vi "ElevatorSystemV2SetState.vi"(1 "Intake Status":T1, 2 "Scoring Deploy Status":cluster{"State":enum16{"Idle", "Deploy"}}, 3 "Elevator Inputs":T2) -> (0 "Elevator Status":T3)   [LabVIEW 2014]
panel:
  in  "Ready to Index?":bool
  # "Low Height"
  # "High Height"
  # "Elevator Motor"
  # "Elevator Encoder"
  # "Proximity Sensor"
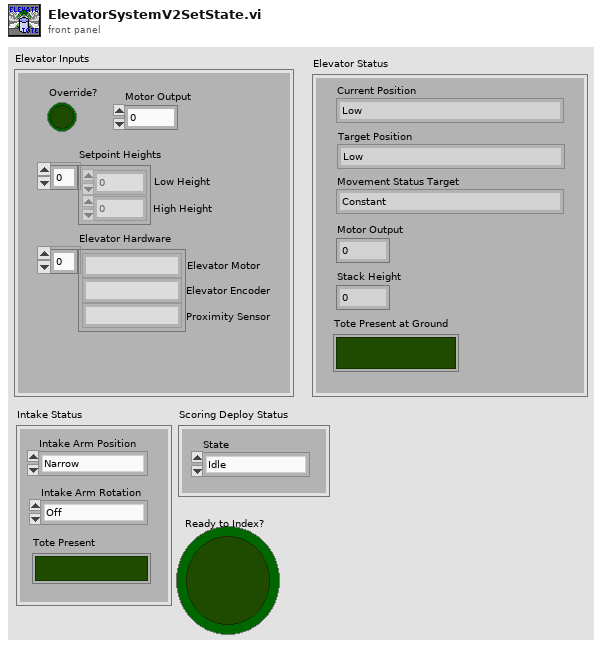
[diagram p1: front panel]
types:
  T1 = cluster{"Intake Arm Position":enum16{"Narrow", "Wide"}, "Intake Arm Rotation":enum16{"Off", "In", "Out", "Rotate Tote"}, "Tote Present":bool}
  T2 = cluster{"Motor Output":dbl, "Override?":bool, "Setpoint Heights":dbl[], "Elevator Hardware":string[]}
  T3 = cluster{"Current Position":enum16{"Low", "High", "Intermediary (Between positions)"}, "Movement Status Target":enum16{"Constant", "Lifting", "Lowering"}, "Stack Height":i32, "Tote Present at Ground":bool, "Target Position":enum16{"Low", "High"}, "Motor Output":dbl}
  T4 = enum16{"Low", "High", "Intermediary (Between positions)"}
  T5 = typedef "WPI_EncoderDevRef.ctl" = cluster{"DevStatus":errorcluster, "EncoderIndex":T6, "CounterIndex":T7, "DistancePerCount":dbl, "Decoding Type":T8}
  T6 = typedef "FPGA_EncoderIdx.ctl" = enum8{"Enc 0", "Enc 1", "Enc 2", "Enc 3", "Enc 4", "Enc 5", "Enc 6", "Enc 7", "Invalid"}
  T7 = typedef "FPGA_CounterCtrSystemIndex.ctl" = enum8{"Ctr 0", "Ctr 1", "Ctr 2", "Ctr 3", "Ctr 4", "Ctr 5", "Ctr 6", "Ctr 7", "Invalid"}
  T8 = typedef "WPI_EncoderType.ctl" = enum16{"1x", "2x", "4x"}
  T9 = typedef "WPI_DigitalInputDevRef.ctl" = cluster{"DevStatus":errorcluster, "DIO Channel":T10, "Controller":T11}
  T10 = typedef "FPGA_DIOChannel.ctl" = enum8{"DIO 0", "DIO 1", "DIO 2", "DIO 3", "DIO 4", "DIO 5", "DIO 6", "DIO 7", "DIO 8", "DIO 9", "DIO MXP 0", "DIO MXP 1", "DIO MXP 2", "DIO MXP 3", "DIO MXP 4", "DIO MXP 5", "DIO MXP 6", "DIO MXP 7", "DIO MXP 8", "DIO MXP 9", "DIO MXP 10", "DIO MXP 11", "DIO MXP 12", "DIO MXP 13", "DIO MXP 14", "DIO MXP 15", "Invalid"}
  T11 = typedef "FPGA_TypedefDigitalModule.ctl" = enum16{"Controller 1"}
  T12 = typedef "WPI_MotorControlDeviceRef.ctl" = cluster{"DeviceStatus":errorcluster, "Type":T13, "PWM":cluster{"Controller":T11, "PWM Channel":T14, "DeadBand":T15}, "CAN":cluster{"Device Number":u8, "Control Mode":T16, "Semaphore":T17, "Max Vout":dbl, "TalonSRX Control Mode":T18}, "Invert":bool, "TransformRef":T19, "InvTransformRef":T19}
  T13 = typedef "WPI_MotorControlType.ctl" = enum16{"PWM", "CAN", "CANTalonSRX"}
  T14 = typedef "FPGA_DIOPWMChannel.ctl" = enum8{"PWM 0", "PWM 1", "PWM 2", "PWM 3", "PWM 4", "PWM 5", "PWM 6", "PWM 7", "PWM 8", "PWM 9", "PWM MXP 0", "PWM MXP 1", "PWM MXP 2", "PWM MXP 3", "PWM MXP 4", "PWM MXP 5", "PWM MXP 6", "PWM MXP 7", "PWM MXP 8", "PWM MXP 9", "Invalid"}
  T15 = typedef "WPI_PWMDeadband.ctl" = cluster{"Name":string, "maxPositivePwm":i32, "minPositivePwm":i32, "centerPwm":i32, "maxNegativePwm":i32, "minNegativePwm":i32, "angularRange":u16}
  T16 = typedef "WPI_CANJaguar_ControlMode.ctl" = enum8{"Percent VBus", "Current", "Speed", "Position", "Voltage"}
  T17 = typedef "Semaphore RefNum" = refnum<k1>
  T18 = typedef "WPI_CANTalonSRX_APIControlMode.ctl" = enum8{"Percent VBus", "Speed", "Position", "Slave", "Unchanged / Invalid"}
  T19 = typedef "WPI_PWMTransform_ConPane.ctl" = refnum<vi>
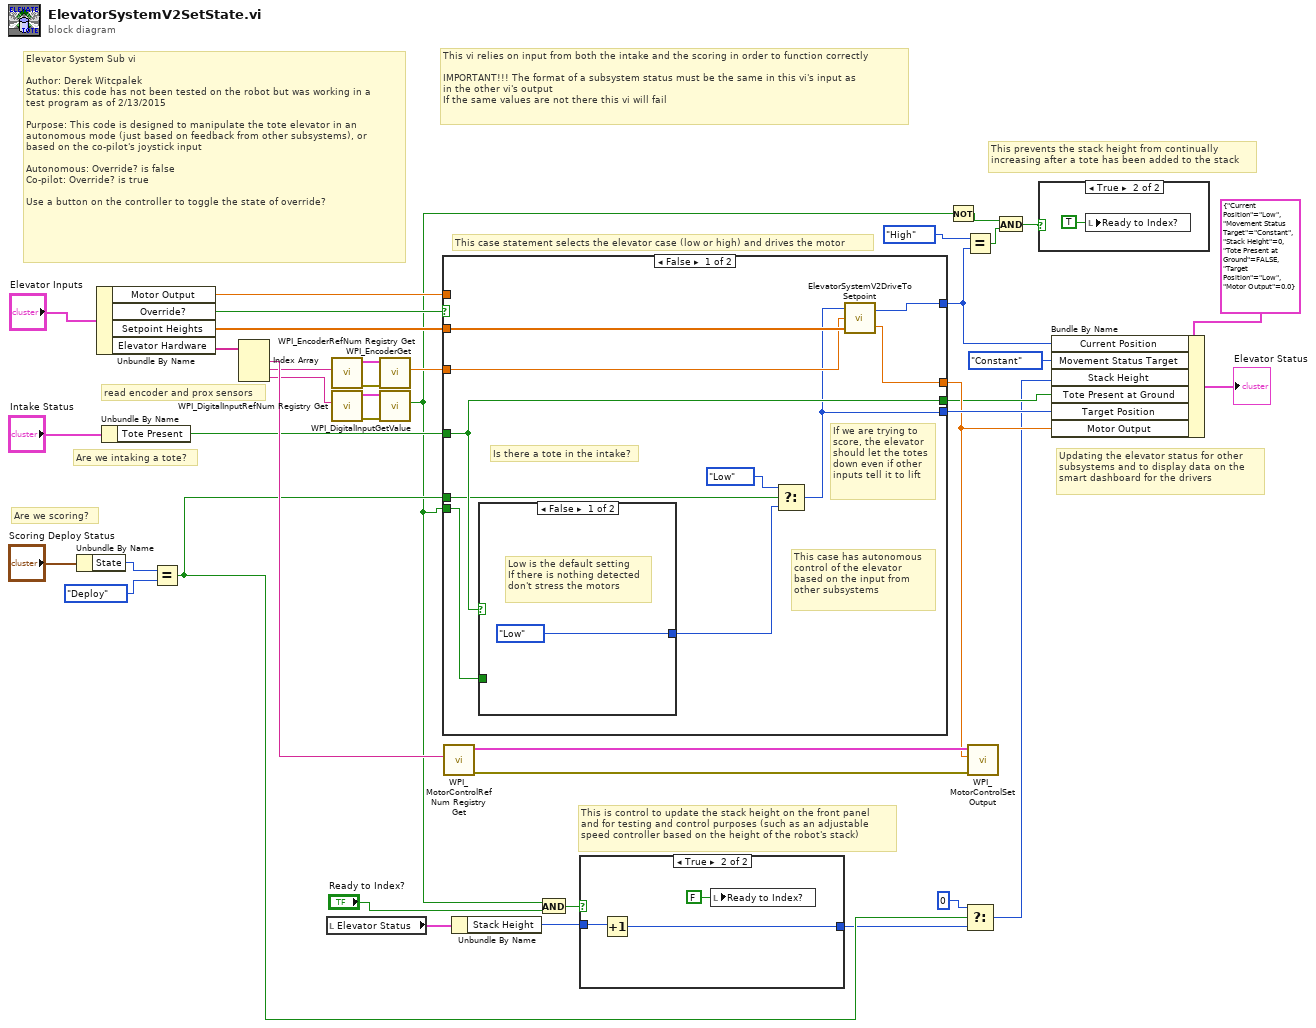
[diagram p0: block diagram]
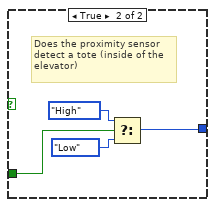
[diagram p4: hidden frame]
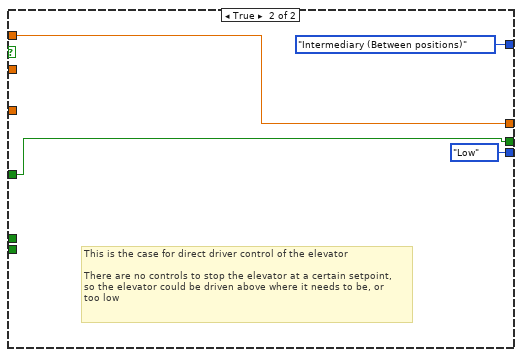
[diagram p5: hidden frame]
diagram:
  # "This vi relies on input from both the intake and the scoring in order to function correctly\n\nIMPORTANT!!! The format of a subsystem status must be the same in this vi's input as\nin the other vi's output\nIf the same values are not there this vi will fail"
  # "Are we intaking a tote?"
  # "Are we scoring?"
  # "read encoder and prox sensors"
  # "Updating the elevator status for other\nsubsystems and to display data on the \nsmart dashboard for the drivers"
  # "This prevents the stack height from continually\nincreasing after a tote has been added to the stack"
  # "This is control to update the stack height on the front panel\nand for testing and control purposes (such as an adjustable \nspeed controller based on the height of the robot's stack)"
  # "This case statement selects the elevator case (low or high) and drives the motor"
  # "Elevator System Sub vi\n\nAuthor: Derek Witcpalek\nStatus: this code has not been tested on the robot but was working in a \ntest program as of 2/13/2015\n\nPurpose: This code is designed to manipulate the tote elevator in an \nautonomous mode (just based on feedback from other subsystems), or \nbased on the co-pilot's joystick input\n\nAutonomous: Override? is false\nCo-pilot: Override? is true\n\nUse a button on the controller to toggle the state of override?"
  n1 = Unbundle By Name("Scoring Deploy Status") -> ("State"=w13:enum16{"Idle", "Deploy"})
  n2 = Unbundle By Name("Elevator Inputs") -> ("Motor Output"=w35:dbl, "Override?"=w39:bool, "Setpoint Heights"=w20:dbl[], "Elevator Hardware"=w21:string[])
  n3 = Unbundle By Name("Intake Status") -> ("Tote Present"=w27:bool)
  n4 = Equal?(x=w13, y=enum16{"Idle", "Deploy"}."Deploy") -> (x = y?=w11:bool)
  n5 = Index Array(array=w21) -> (element #1=w38:string, element #2=w33:string, element #3=w34:string)  [unwired: 3 in]
  n6 = local read "Elevator Status"() -> (w16:T3)
  n7 = call <vilib>:"WPI_EncoderRefNum Registry Get.vi"("refnum name"=w33) -> ("error out"=w32:errorcluster, "EncoderDevRef"=w31:T5)  [unwired: 9 in]
  n8 = call <vilib>:"WPI_DigitalInputRefNum Registry Get.vi"("refnum name"=w34) -> ("error out"=w30:errorcluster, "DigitalInputDevRef"=w29:T9)  [unwired: 9 in]
  n9 = call <vilib>:"WPI_EncoderGet.vi"("error in (no error)"=w32, "EncoderDevRef"=w31) -> ("Distance"=w19:dbl)  [unwired: 4 in, 5 out]
  n10 = call <vilib>:"WPI_DigitalInputGetValue.vi"("error in (no error)"=w30, "DigitalInputDevRef"=w29) -> ("Value"=w5:bool)  [unwired: 7 in, 2 out]
  n11 = case shown="False" w39 {
    tunnel: [w49 w59] -> w23
    tunnel: w35 -> [_ w59]
    tunnel: w27 -> [w45 w56]
    tunnel: [w41 enum16{"Low", "High"}."Low" ("f")] -> w24
    tunnel: w5 -> [w50 _]
    tunnel: [w48 T4."Intermediary (Between positions)" ("Current Position")] -> w3
    tunnel: w20 -> [w47 _]
    tunnel: w19 -> [w46 _]
    tunnel: [w45 w56] -> w18
    tunnel: w11 -> [w43 _]
    frame False {
      # "If we are trying to\nscore, the elevator\nshould let the totes\ndown even if other\ninputs tell it to lift"
      # "Is there a tote in the intake?"
      # "This case has autonomous\ncontrol of the elevator \nbased on the input from\nother subsystems"
      n12 = case shown="False" w45 {
        tunnel: [enum16{"Low", "High"}."Low" ("Target Position") w55] -> w44
        tunnel: w50 -> [_ w54]
        frame False {
          # "Low is the default setting\nIf there is nothing detected\ndon't stress the motors"
        }
        frame True {
          # "Does the proximity sensor\ndetect a tote (inside of the \nelevator)"
          n13 = Select(t=enum16{"Low", "High"}."High" ("Target Position"), s=w54, f=enum16{"Low", "High"}."Low") -> (s? t:f=w55:enum16{"Low", "High"})
        }
      }
      n14 = Select(t=enum16{"Low", "High"}."Low", s=w43, f=w44) -> (s? t:f=w41:enum16{"Low", "High"})
      n15 = call "ElevatorSystemV2DriveToSetpoint.vi"("Setpoints"=w47, "Encoder Reading"=w46, "Target Position"=w41) -> ("Motor Output"=w49:dbl, "Current Position"=w48:T4)
    }
    frame True {
      # "This is the case for direct driver control of the elevator\n\nThere are no controls to stop the elevator at a certain setpoint,\nso the elevator could be driven above where it needs to be, or \ntoo low"
    }
  }
  n16 = call <vilib>:"WPI_MotorControlRefNum Registry Get.vi"("refnum name"=w38) -> ("error out"=w36:errorcluster, "MotorControlDevRef"=w37:T12)  [unwired: 9 in]
  n17 = Unbundle By Name(w16) -> ("Stack Height"=w15:i32)
  n18 = And(x=w5, y="Ready to Index?") -> (x .and. y?=w17:bool)
  n19 = case shown="True" w17 {
    tunnel: w15 -> [w60 w62]
    tunnel: [w60 w61] -> w10
    frame False {
    }
    frame True {
      n20 = Increment(x=w62) -> (x+1=w61:i32)
      n21 = local write "Ready to Index?"(FALSE ("Ready to Index?")) -> ()
    }
  }
  n22 = Not(x=w5) -> (.not. x?=w6:bool)
  n23 = Equal?(x=T4."High", y=w3) -> (x = y?=w4:bool)
  n24 = Select(t=0, s=w11, f=w10) -> (s? t:f=w8:i32)
  n25 = call <vilib>:"WPI_MotorControlSetOutput.vi"("error in (no error)"=w36, "Output"=w23, "MotorControlDevRef"=w37) -> ()  [unwired: 6 in, 3 out]
  n26 = And(x=w6, y=w4) -> (x .and. y?=w7:bool)
  n27 = case shown="True" w7 {
    frame False {
    }
    frame True {
      n28 = local write "Ready to Index?"(TRUE ("Ready to Index?")) -> ()
    }
  }
  n29 = Bundle By Name(cluster=T3 {"Current Position"=enum."Low", "Movement Status Target"=enum."Constant", "Stack Height"=0, "Tote Present at Ground"=FALSE, "Target Position"=enum."Low", "Motor Output"=0.0} ("Elevator Status 2"), "Current Position"=w3, "Movement Status Target"=enum16{"Constant", "Lifting", "Lowering"}."Constant", "Stack Height"=w8, "Tote Present at Ground"=w18, "Target Position"=w24, "Motor Output"=w23) -> (→"Elevator Status":T3)
